vi "Error Query (Multiple).vi"(8 "error in (no error)":errorcluster, 11 "VISA Resource Name":refnum<visa-resource-name>) -> (0 "error out":errorcluster, 1 "error message":string, 2 "error":bool, 3 "VISA Resource Name Out":refnum<visa-resource-name>)   [LabVIEW 2010, in "Tektronix TDS 3000 Series.lvlib"]
doc: "This VI reads the error queue from the instrument. It expects to see errors in SCPI format (#,\"error message\"). It continues to read from the error queue until it reads a 0, \"No error\"."
uses:
  <instrlib>/Tektronix TDS 3000 Series/Tektronix TDS 3000 Series.lvlib
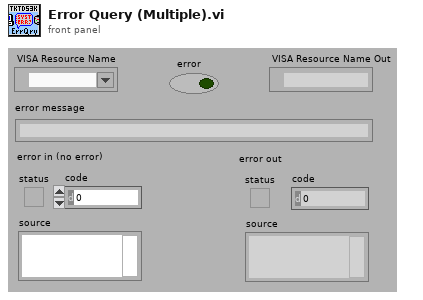
[diagram p1: front panel]
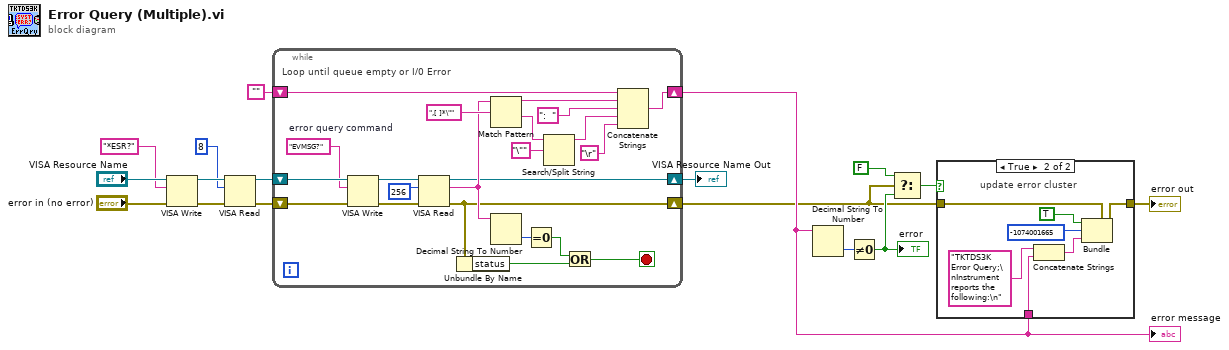
[diagram p0: block diagram]
diagram:
  n1 = VISA Write(VISA resource name="VISA Resource Name", write buffer="*ESR?" ("Command"), error in (no error)="error in (no error)") -> (VISA resource name out=w7:refnum<visa-resource-name>, error out=w6:errorcluster)  [unwired: 1 out]
  n2 = VISA Read(VISA resource name=w7, byte count=u32 8 ("byte count (0)"), error in (no error)=w6) -> (VISA resource name out=w9:refnum<visa-resource-name>, error out=w8:errorcluster)  [unwired: 2 out]
  n3 = while {
    shift-left: w9 -> [w37]
    shift-right: [w23] -> w16
    shift-left: w8 -> [w38]
    shift-right: [w24] -> w1
    shift-left: "" -> [w39]
    shift-right: [w22] -> w14
    stop <- w18 stop-if-true
    w32 = "EVMSG?"  # error query command
    # "Loop until queue empty or I/0 Error"
    n4 = VISA Write(VISA resource name=w37, write buffer=w32, error in (no error)=w38) -> (VISA resource name out=w31:refnum<visa-resource-name>, error out=w30:errorcluster)  [unwired: 1 out]
    n5 = VISA Read(VISA resource name=w31, byte count=u32 256, error in (no error)=w30) -> (VISA resource name out=w23:refnum<visa-resource-name>, read buffer=w25:string, error out=w24:errorcluster)  [unwired: 1 out]
    n6 = Unbundle By Name(w24) -> ("status"=w34:bool)
    n7 = Match Pattern(string=w25, regular expression=",[ ]*\"") -> (before substring=w28:string, after substring=w26:string)  [unwired: 1 in, 2 out]
    n8 = Decimal String To Number(string=w25) -> (number=w36:i32)  [unwired: 2 in, 1 out]
    n9 = Equal To 0?(x=w36) -> (x = 0?=w35:bool)
    n10 = Search/Split String(string=w26, search string/char (-)="\"") -> (substring before match=w20:string)  [unwired: 1 in, 2 out]
    n11 = Or(x=w35, y=w34) -> (x .or. y?=w18:bool)
    n12 = Concatenate Strings(w39, w28, ":  ", w20, "\r") -> (w22:string)
  }
  "error message" <- w14
  "VISA Resource Name Out" <- w16
  n13 = Decimal String To Number(string=w14) -> (number=w15:i32)  [unwired: 2 in, 1 out]
  n14 = Not Equal To 0?(x=w15) -> (x != 0?=w11:bool)
  "error" <- w11
  n15 = Select(t=FALSE, s=w1, f=w11) -> (s? t:f=w10:bool)
  n16 = case shown="True" w10 {
    tunnel: w1 -> [w40 w45]
    tunnel: [w40 w44] -> w13
    tunnel: w14 -> [_ w41]
    frame False {
      # "no instrument errors"
    }
    frame True {
      # "update error cluster"
      n17 = Concatenate Strings("TKTDS3K Error Query;\nInstrument reports the following:\n", w41) -> (w43:string)
      n18 = Bundle(cluster=w45, "status"=TRUE, "code"=-1074001665, "source"=w43) -> (w44:errorcluster)
    }
  }
  "error out" <- w13
